vi "ProgG_006_MG.vi"() -> ()   [LabVIEW 2021]
panel:
  out "Y":dbl=14.105
  in  "x2":ext=19.4
  in  "x1":ext=14.1
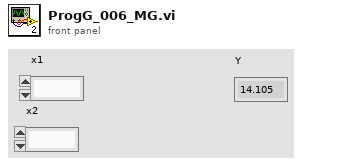
[diagram p1: front panel]
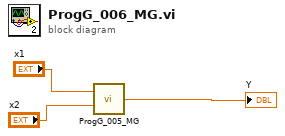
[diagram p0: block diagram]
diagram:
  n1 = call "ProgG_005_MG.vi"("x2"="x2", "x1"="x1") -> ("Y"=→"Y":dbl)
